vi "utility.String to Array.vi"(1 "命令输入":string) -> (0 "输出数组":u8[](array[numeric]) format="%02x")   [LabVIEW 2012, in "Lib_UEL.ATE.lvlib" / "Lib_App.lvlib"]
uses:
  Lib_App.lvlib
panel:
  out "空格数":i32=2
  out "最终数组":string[](array[string])
  out "2合1":string
  out "转置数组":string[](array[string])
  out "无符号字节数组":u8[](array[numeric])
  # "功能:\n1.转换字符串到V8数值数组;忽略非(0-F)字符;\n2.转换方式\n  - 每两个字符对应一个V8数值;\n  - 以空格,',',';','|','-'为分隔符,转换字符到V8数值;\n  - 如果只有一个字符,则作为V8数值的低位;"
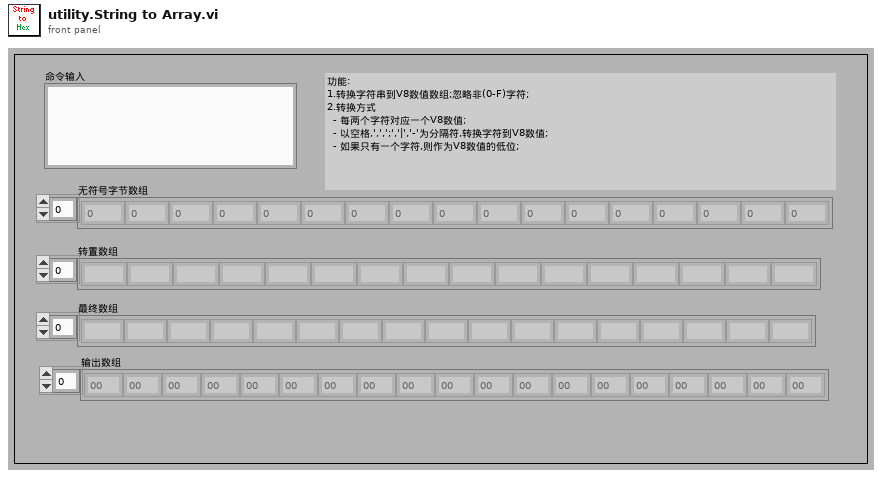
[diagram p1: front panel]
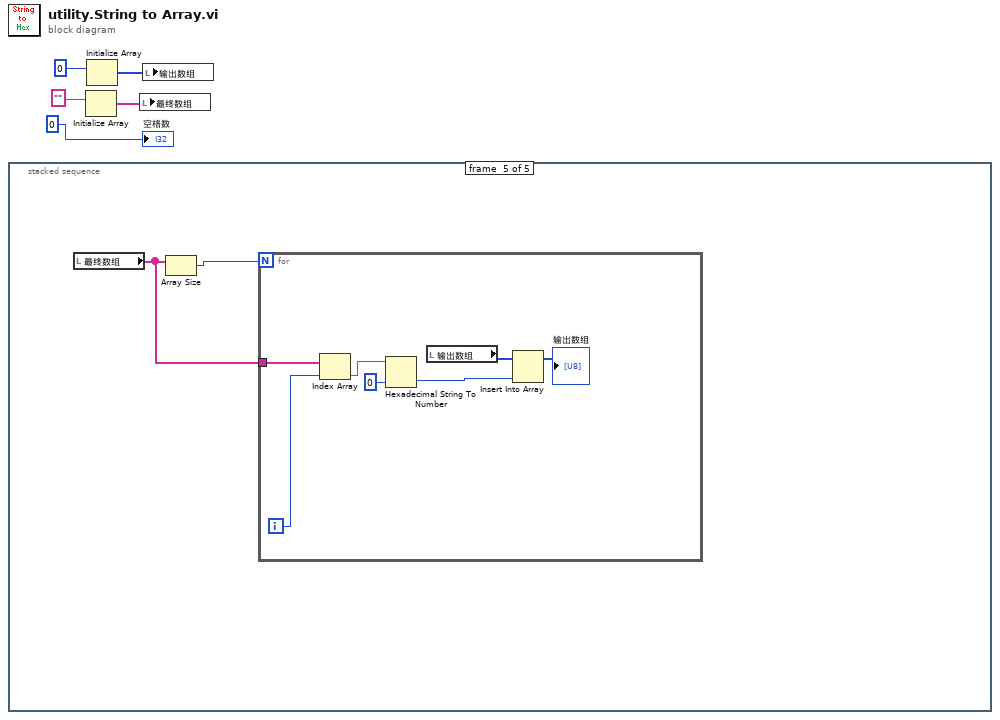
[diagram p0: block diagram]
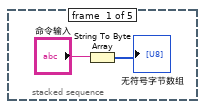
[diagram p2: hidden frame]
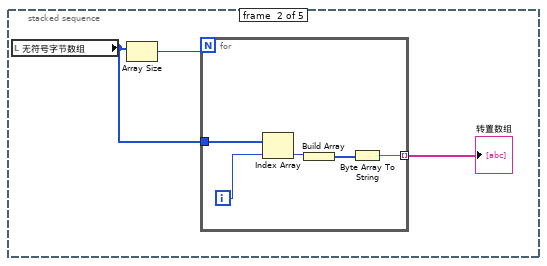
[diagram p3: hidden frame]
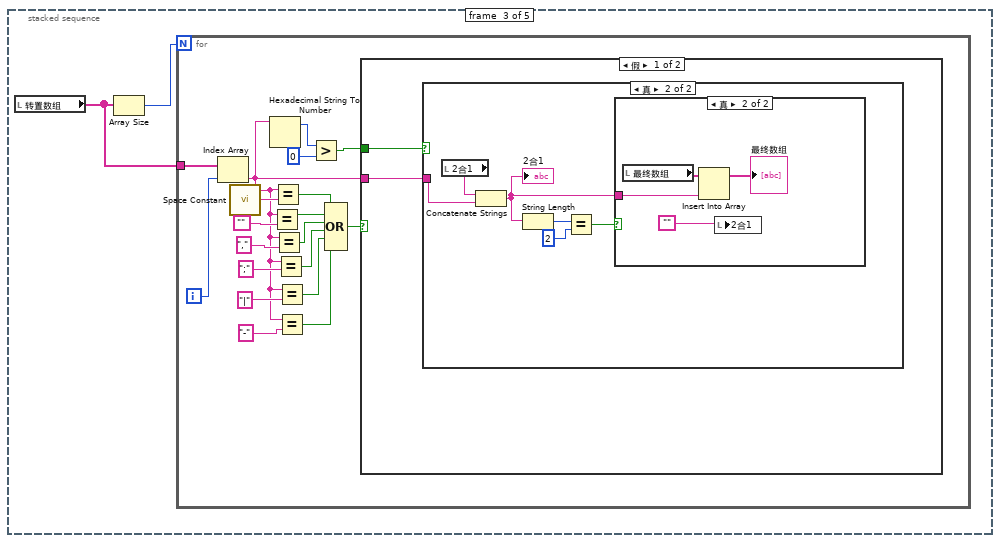
[diagram p4: hidden frame]
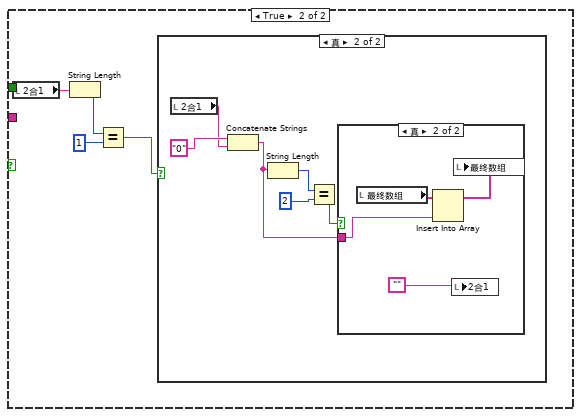
[diagram p7: hidden frame]
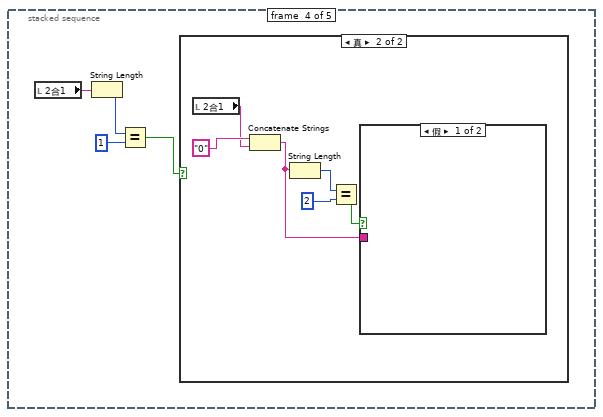
[diagram p10: hidden frame]
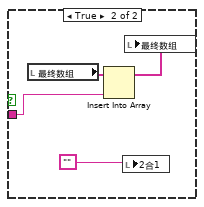
[diagram p12: hidden frame]
diagram:
  n1 = stacked-sequence {
    frame #0 {
      n2 = String To Byte Array(string="命令输入") -> (unsigned byte array=→"无符号字节数组":u8[])
    }
    frame #1 {
      n3 = local read "无符号字节数组"() -> (w9:u8[])
      n4 = Array Size(array=w9) -> (size(s)=w10:i32)
      n5 = for {
        N: w10 -> [_]
        tunnel: w9 -> [w15]
        tunnel: [w11] -> w8 mode=indexing
        i -> [w14]
        n6 = Index Array(array=w15, index=w14) -> (element=w13:u8)
        n7 = Build Array(w13) -> (w12:u8[])
        n8 = Byte Array To String(unsigned byte array=w12) -> (string=w11:string)
      }
      "转置数组" <- w8
    }
    frame #2 {
      n9 = local read "转置数组"() -> (w16:string[])
      n10 = Array Size(array=w16) -> (size(s)=w17:i32)
      n11 = for {
        N: w17 -> [_]
        tunnel: w16 -> [w36]
        i -> [w35]
        n12 = Index Array(array=w36, index=w35) -> (element=w21:string)
        n13 = call <vilib>:"Space Constant.vi"() -> ("String"=w34:string)
        n14 = Hexadecimal String To Number(string=w21) -> (offset past number=w20:i32)  [unwired: 2 in, 1 out]
        n15 = Equal?(x=w21, y="") -> (x = y?=w31:bool)
        n16 = Equal?(x=w21, y=w34) -> (x = y?=w32:bool)
        n17 = Equal?(x=w21, y=",") -> (x = y?=w25:bool)
        n18 = Equal?(x=w21, y=";") -> (x = y?=w24:bool)
        n19 = Equal?(x=w21, y="|") -> (x = y?=w23:bool)
        n20 = Equal?(x=w21, y="-") -> (x = y?=w22:bool)
        n21 = Greater?(x=w20, y=0) -> (0:w18:bool)
        n22 = Compound Arithmetic op=OR(w32, w31, w25, w24, w23, w22) -> (w30:bool)
        n23 = case shown="假" w30 {
          tunnel: w21 -> [w38 _]
          tunnel: w18 -> [w37 _]
          frame False {
            n24 = case shown="真" w37 {
              tunnel: w38 -> [_ w40]
              frame False {
              }
              frame True {
                n25 = local read "2合1"() -> (w39:string)
                n26 = Concatenate Strings(w39, w40) -> (w41:string)
                "2合1" <- w41
                n27 = String Length(string=w41) -> (length=w44:i32)
                n28 = Equal?(x=w44, y=2) -> (x = y?=w42:bool)
                n29 = case shown="真" w42 {
                  tunnel: w41 -> [_ w48]
                  frame False {
                  }
                  frame True {
                    n30 = local read "最终数组"() -> (w46:string[])
                    n31 = Insert Into Array(array=w46, new element=w48) -> (→"最终数组":string[])  [unwired: 1 in]
                    n32 = local write "2合1"("") -> ()
                  }
                }
              }
            }
          }
          frame True {
            n33 = local read "2合1"() -> (w52:string)
            n34 = String Length(string=w52) -> (length=w51:i32)
            n35 = Equal?(x=w51, y=1) -> (x = y?=w49:bool)
            n36 = case shown="真" w49 {
              frame False {
              }
              frame True {
                n37 = local read "2合1"() -> (w53:string)
                n38 = Concatenate Strings("0", w53) -> (w55:string)
                n39 = String Length(string=w55) -> (length=w58:i32)
                n40 = Equal?(x=w58, y=2) -> (x = y?=w56:bool)
                n41 = case shown="真" w56 {
                  tunnel: w55 -> [_ w61]
                  frame False {
                  }
                  frame True {
                    n42 = local read "最终数组"() -> (w62:string[])
                    n43 = Insert Into Array(array=w62, new element=w61) -> (w60:string[])  [unwired: 1 in]
                    n44 = local write "2合1"("") -> ()
                    n45 = local write "最终数组"(w60) -> ()
                  }
                }
              }
            }
          }
        }
      }
    }
    frame #3 {
      n46 = local read "2合1"() -> (w66:string)
      n47 = String Length(string=w66) -> (length=w65:i32)
      n48 = Equal?(x=w65, y=1) -> (x = y?=w63:bool)
      n49 = case shown="真" w63 {
        frame False {
        }
        frame True {
          n50 = local read "2合1"() -> (w67:string)
          n51 = Concatenate Strings("0", w67) -> (w69:string)
          n52 = String Length(string=w69) -> (length=w72:i32)
          n53 = Equal?(x=w72, y=2) -> (x = y?=w70:bool)
          n54 = case shown="假" w70 {
            tunnel: w69 -> [_ w75]
            frame False {
            }
            frame True {
              n55 = local read "最终数组"() -> (w76:string[])
              n56 = Insert Into Array(array=w76, new element=w75) -> (w74:string[])  [unwired: 1 in]
              n57 = local write "2合1"("") -> ()
              n58 = local write "最终数组"(w74) -> ()
            }
          }
        }
      }
    }
    frame #4 {
      n59 = local read "最终数组"() -> (w77:string[])
      n60 = Array Size(array=w77) -> (size(s)=w78:i32)
      n61 = for {
        N: w78 -> [_]
        tunnel: w77 -> [w85]
        i -> [w84]
        n62 = Index Array(array=w85, index=w84) -> (element=w81:string)
        n63 = Hexadecimal String To Number(string=w81, default (0uL)=u8 0 ("默认(0 U32)")) -> (number=w80:u8)  [unwired: 1 in, 1 out]
        n64 = local read "输出数组"() -> (w82:u8[])
        n65 = Insert Into Array(array=w82, new element=w80) -> (→"输出数组":u8[])  [unwired: 1 in]
      }
    }
  }
  n66 = Initialize Array("") -> (w4:string[])  [unwired: 1 in]
  n67 = Initialize Array(0) -> (w2:i32[])  [unwired: 1 in]
  n68 = local write "最终数组"(w4) -> ()
  n69 = local write "输出数组"(w2) -> ()
  "空格数" <- 0
